vi "Check Linked Node.vi"(6 "Use Channel?":bool, 8 "error in (no error)":errorcluster, 9 "NodeName":string, 11 "Item Ref in":T1 format="%.0x") -> (0 "error out":errorcluster, 3 "Item Ref out":T1 format="%.0x")   [LabVIEW 2015, in "Control Addon System Explorer.lvlib"]
uses:
  Control Addon System Explorer.lvlib
  <vilib>/NI Veristand/Custom Device API/Custom Device Item Ref.ctl
  NationalInstruments.VeriStand.SystemStorage
  <vilib>/NI Veristand/Custom Device API/Get Item Property (Dependent Node Pointer).vi
  <vilib>/NI VeriStand/Custom Device API/Custom Device API.lvlib
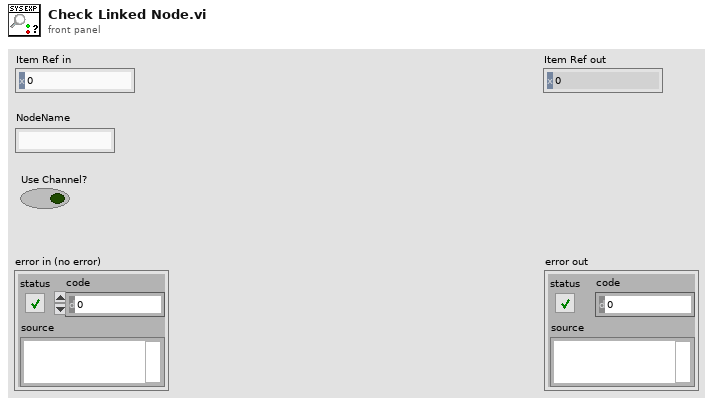
[diagram p1: front panel]
types:
  T1 = typedef "Custom Device API.lvlib/Custom Device Item Ref.ctl" = u64
  T2 = typedef "Custom Device API.lvlib/Custom Device Pointer.ctl" = refnum<k24>
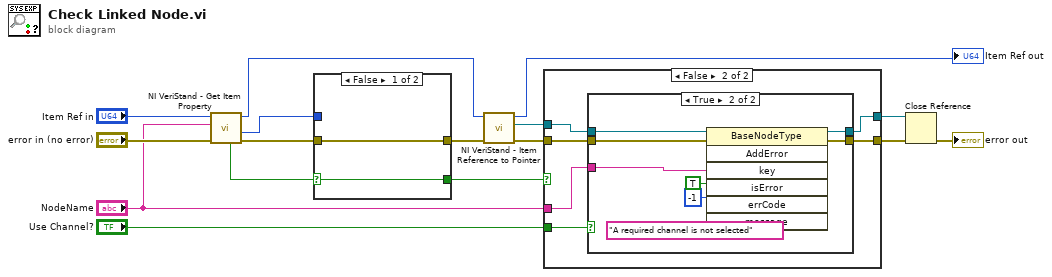
[diagram p0: block diagram]
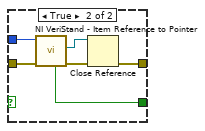
[diagram p2: hidden frame]
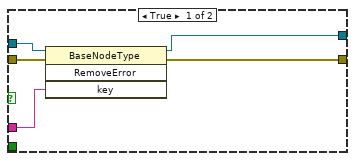
[diagram p3: hidden frame]
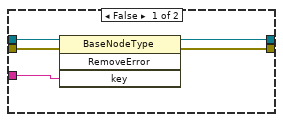
[diagram p4: hidden frame]
diagram:
  n1 = call-poly <vilib>:"NI VeriStand - Get Item Property.vi"("error in (no error)"="error in (no error)", "Property Name"="NodeName", "Item Ref in"="Item Ref in") -> ("error out"=w6:errorcluster, "Dependent Node Ref"=w7:T1, "Item Ref out"=w11:T1, "Found"=w5:bool)  [unwired: 5 in]
  n2 = case shown="False" w5 {
    selector: w5 -> [w16 _]
    tunnel: w7 -> [_ w23]
    tunnel: w6 -> [w17 w22]
    tunnel: [w17 w21] -> w2
    tunnel: [w16 w20] -> w3
    frame False {
    }
    frame True {
      n3 = call <vilib>:"NI VeriStand - Item Reference to Pointer.vi"("error in (no error)"=w22, "Item Ref in"=w23) -> ("error out"=w19:errorcluster, "Node Pointer"=w18:T2, "Found"=w20:bool)  [unwired: 6 in, 1 out]
      n4 = Close Reference(reference=w18, error in (no error)=w19) -> (error out=w21:errorcluster)
    }
  }
  n5 = call <vilib>:"NI VeriStand - Item Reference to Pointer.vi"("error in (no error)"=w2, "Item Ref in"=w11) -> ("Node Pointer"=w14:T2, "Item Ref out"=→"Item Ref out":T1)  [unwired: 6 in, 2 out]
  n6 = case shown="False" w3 {
    tunnel: [w28 w34] -> w4
    tunnel: w2 -> [w24 w29]
    tunnel: "Use Channel?" -> [_ w33]
    tunnel: w14 -> [w27 w32]
    tunnel: [w26 w31] -> w13
    tunnel: "NodeName" -> [w25 w30]
    frame True {
      n7 = invoke class="BaseNodeType" method="RemoveError"(reference=w27, error in=w24, "key"=w25) -> (reference out=w26:T2, error out=w28:errorcluster)  [unwired: 1 in, 2 out]
    }
    frame False {
      n8 = case shown="True" w33 {
        tunnel: w29 -> [w39 w43]
        tunnel: [w38 w47] -> w34
        tunnel: w32 -> [w37 w44]
        tunnel: [w36 w41] -> w31
        tunnel: w30 -> [w35 w40]
        frame False {
          n9 = invoke class="BaseNodeType" method="RemoveError"(reference=w37, error in=w39, "key"=w35) -> (reference out=w36:T2, error out=w38:errorcluster)  [unwired: 1 in, 2 out]
        }
        frame True {
          n10 = invoke class="BaseNodeType" method="AddError"(reference=w44, error in=w43, "key"=w40, "isError"=TRUE, "errCode"=-1, "message"="A required channel is not selected") -> (reference out=w41:T2, error out=w47:errorcluster)  [unwired: 1 in, 5 out]
        }
      }
    }
  }
  n11 = Close Reference(reference=w13, error in (no error)=w4) -> (error out=→"error out":errorcluster)
